vi "Send ConnectionDied.vi"(7 "Message Priority (Normal)":T1=enum."Normal", 8 "error in (no error)":errorcluster, 10 "Connection":refnum<class "Connection.lvclass">, 11 "Message Enqueuer":refnum<class "Message Enqueuer.lvclass">) -> (0 "error out":errorcluster, 3 "Message Enqueuer out":refnum<class "Message Enqueuer.lvclass">)   [LabVIEW 2022 SP3, in "Connection.lvlib" / "ConnectionDied Msg.lvclass"]
doc: "This VI sends the message to an actor."
uses:
  ConnectionDied Msg.lvclass
  <vilib>/ActorFramework/Message Enqueuer/Message Enqueuer.lvclass
  C:/Program Files (x86)/National Instruments/LabVIEW 2022/vi.lib/ActorFramework/Message/Message.lvclass
  C:/Users/jakub/repos/gh/lv-cli-example/Source/Connection/CallerMessage Messages/ConnectionDied Msg/ConnectionDied Msg.lvclass
  <vilib>/ActorFramework/Message Enqueuer/Message Priority.ctl
  TcpSocket/Source/TcpSocket/Connection/Connection.lvclass
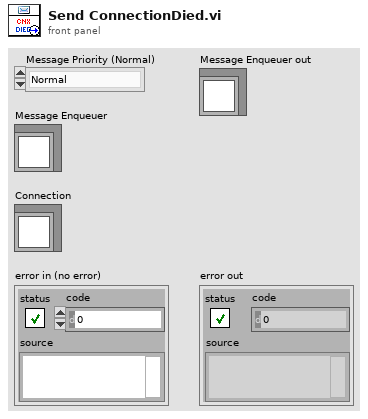
[diagram p1: front panel]
types:
  T1 = typedef "Actor Framework.lvlib/Message Enqueuer.lvclass/Message Priority.ctl" = enum16{"Low", "Normal", "High"}
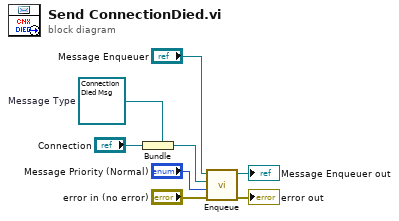
[diagram p0: block diagram]
diagram:
  w5 = refnum<class "ConnectionDied Msg.lvclass"> refnum  # Message Type
  n1 = Bundle(cluster=w5, "Connection") -> (w4:refnum<class "ConnectionDied Msg.lvclass">)
  n2 = call <vilib>:"Enqueue.vi"("error in (no error)"="error in (no error)", "Message Priority (Normal)"="Message Priority (Normal)", "Message"=w4, "Message Enqueuer in"="Message Enqueuer") -> ("error out"=→"error out":errorcluster, "Message Enqueuer out"=→"Message Enqueuer out":refnum<class "Message Enqueuer.lvclass">)  [unwired: 6 in]
